vi "Find Zero.vi"(11 "Circular Buffer in":refnum<class "Circular Buffer.lvclass">) -> (3 "Circular Buffer out":refnum<class "Circular Buffer.lvclass">)   [LabVIEW 2023, in "d20.lvlib" / "Circular Buffer.lvclass"]
uses:
  Circular Buffer.lvclass
  Circular Buffer.lvclass/Circular Buffer.ctl
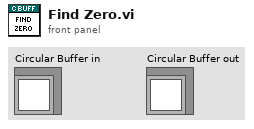
[diagram p1: front panel]
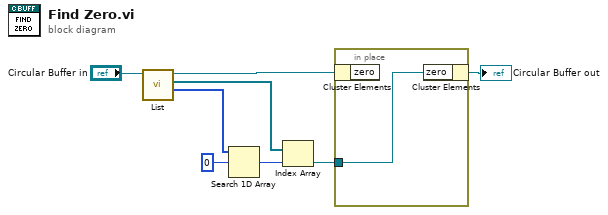
[diagram p0: block diagram]
diagram:
  n1 = call "List.vi"("Circular Buffer in"="Circular Buffer in") -> ("Shift List"=w6:i64[], "Node List"=w7:refnum<data-value>[], "Circular Buffer out"=w2:refnum<class "Circular Buffer.lvclass">)  [unwired: 7 in, 1 out]
  n2 = Search 1D Array(1D array=w6, element=0) -> (index of element=w8:i32)  [unwired: 1 in]
  n3 = Index Array(array=w7, index=w8) -> (element=w3:refnum<data-value>)
  n4 = in-place {
    in-place-border: w3 -> [w9]
    n5 = in-place-cluster #1(w2) -> ()  [unwired: 1 out]
    n6 = in-place-cluster #1("zero"=w9) -> (→"Circular Buffer out":refnum<class "Circular Buffer.lvclass">)
  }
